vi "Fetch (Multiple Binary Data).vi"(4 "Buffer Element2":i32(ring) items=["", "Date", "Extra", "Formatted", "Fractional", "Reading", "Relative", "Seconds", "Status", "Time", "Tstamp", "Unit", "CHAN", "Extra Form", "Extra Unit"], 5 "End Index (10)":i32=10, 6 "Buffer Element1":i32(ring) items=["", "Date", "Extra", "Formatted", "Fractional", "Reading", "Relative", "Seconds", "Status", "Time", "Tstamp", "Unit", "CHAN", "Extra Format", "Extra Unit"], 7 "Timeout (100000 ms)":i32=100000, 8 "error in (no error)":errorcluster, 9 "Buffer Name":string, 10 "Start Index (1)":i32=1, 11 "VISA resource name":refnum<visa-resource-name>) -> (0 "error out":errorcluster, 2 "Measurements":sgl[](array[numeric]), 3 "VISA resource name out":refnum<visa-resource-name>)   [LabVIEW 2015, in "Keithley DMM6500 DAQ6500 Series.lvlib"]
doc: "Reads and returns multiple measurements from the instrument. The data are extracted in binary format then converted to Single format measurements. Use this VI when you want to take multiple measurements using an immediate trigger. Use the low-level VIs for other triggering options."
uses:
  <instrlib>/Keithley DMM6500 DAQ6500 Series/Keithley DMM6500 DAQ6500 Series.lvlib
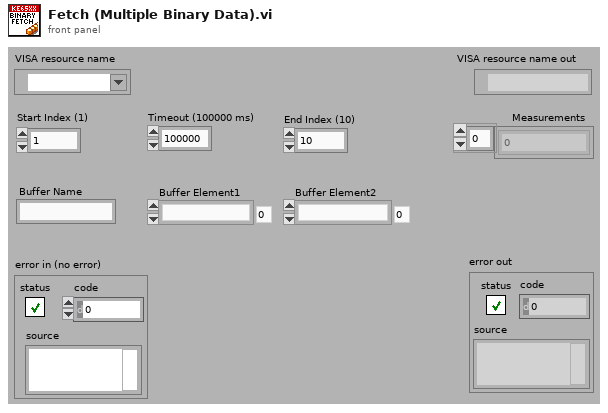
[diagram p1: front panel]
types:
  T1 = enum16{"big-endian, network order", "native, host order", "little-endian"}
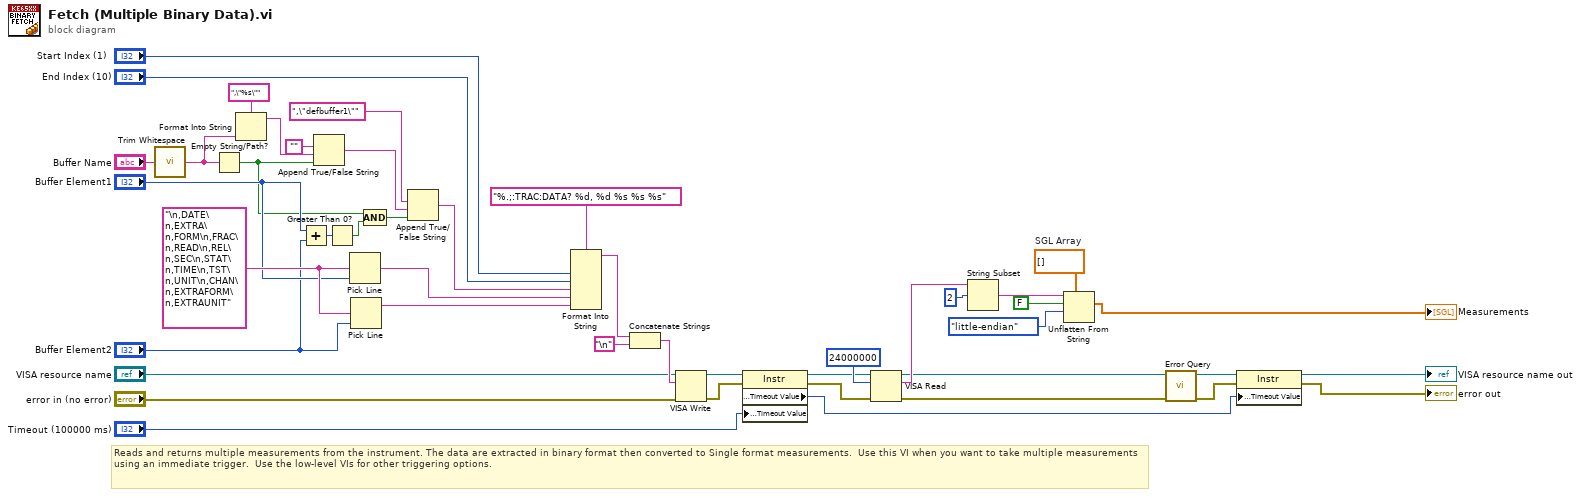
[diagram p0: block diagram]
diagram:
  w6 = sgl[] []  # SGL Array
  w21 = "\n,DATE\n,EXTRA\n,FORM\n,FRAC\n,READ\n,REL\n,SEC\n,STAT\n,TIME\n,TST\n,UNIT\n,CHAN\n,EXTRAFORM\n,EXTRAUNIT" ("multi-line string")
  # "Reads and returns multiple measurements from the instrument. The data are extracted in binary format then converted to Single format measurements.  Use this VI when you want to take multiple measurements using an immediate trigger.  Use the low-level VIs for other triggering options."
  n1 = call <vilib>:"Trim Whitespace.vi"("string"="Buffer Name") -> ("trimmed string"=w12:string)  [unwired: 1 in]
  n2 = Empty String/Path?(string/path=w12) -> (empty?=w11:bool)
  n3 = Format Into String(format string=",\"%s\"", w12) -> (resulting string=w41:string)  [unwired: 2 in, 1 out]
  n4 = Add(x="Buffer Element1", y="Buffer Element2") -> (x+y=w14:i32)
  n5 = Append True/False String(1:w11, 2:w41, 3:"") -> (0:w16:string)  [unwired: 1 in]
  n6 = Greater Than 0?(x=w14) -> (x > 0?=w13:bool)
  n7 = Pick Line(multi-line string=w21, line index="Buffer Element1") -> (output string=w23:string)  [unwired: 1 in]
  n8 = Pick Line(multi-line string=w21, line index="Buffer Element2") -> (output string=w22:string)  [unwired: 1 in]
  n9 = Compound Arithmetic op=AND(w11, w13) -> (w17:bool)
  n10 = Append True/False String(1:w17, 2:w16, 3:",\"defbuffer1\"" ("true string")) -> (0:w18:string)  [unwired: 1 in]
  n11 = Format Into String(format string="%.;:TRAC:DATA? %d, %d %s %s %s", "Start Index (1)", "End Index (10)", w18, w23, w22) -> (resulting string=w29:string)  [unwired: 2 in, 1 out]
  n12 = Concatenate Strings(w29, "\n") -> (w44:string)
  n13 = VISA Write(VISA resource name="VISA resource name", write buffer=w44, error in (no error)="error in (no error)") -> (VISA resource name out=w39:refnum<visa-resource-name>, error out=w38:errorcluster)  [unwired: 1 out]
  n14 = property on="Property Node" class="Instr"(reference=w39, error in=w38, "General Settings:Timeout Value"="Timeout (100000 ms)") -> (reference out=w36:refnum<visa-resource-name>, error out=w37:errorcluster, "General Settings:Timeout Value"=w31:u32)
  n15 = VISA Read(VISA resource name=w36, byte count=i64 24000000, error in (no error)=w37) -> (VISA resource name out=w2:refnum<visa-resource-name>, read buffer=w10:string, error out=w1:errorcluster)  [unwired: 1 out]
  n16 = String Subset(string=w10, offset (0)=2) -> (substring=w3:string)  [unwired: 1 in]
  n17 = Unflatten From String(type=w6, binary string=w3, data includes array or string size? (T)=FALSE, byte order (0:big-endian, network order)=T1."little-endian") -> (value=→"Measurements":sgl[])  [unwired: 1 in, 2 out]
  n18 = call <instrlib>:"Error Query.vi"("error in (no error)"=w1, "VISA resource name"=w2) -> ("error out"=w33:errorcluster, "VISA resource name out"=w35:refnum<visa-resource-name>)  [unwired: 6 in, 2 out]
  n19 = property on="Property Node" class="Instr"(reference=w35, error in=w33, "General Settings:Timeout Value"=w31) -> (reference out=→"VISA resource name out":refnum<visa-resource-name>, error out=→"error out":errorcluster)
